vi "to string.vi"(8 "error in":errorcluster, 11 "Instrument configuration":refnum<class "Instrument configuration.lvclass">) -> (0 "error out":errorcluster, 1 "data":string, 2 "version":string, 3 "Instrument configuration out":refnum<class "Instrument configuration.lvclass">)   [LabVIEW 2025, in "Abstract Engine.lvlib" / "Instrument configuration.lvclass"]
doc: "Provides an interface for saving a module configuration to a file or other serialized data source. It is recommended that all children of this class store data in two sets--data required for its own initialization, and any data required for parent initialization--and that each implementation uses the <b>Call Parent Method</b> primitive to serialize parent information.Copyright 2017 National Instruments Corporation\n\nLicensed under the Apache License, Version 2.0 (the \"License\"); you may not use this file except in compliance with the License. You may obtain a copy of the License at http://www.apache.org/licenses/LICENSE-2.0\nUnless required by applicable law or agreed to in writing, software distributed under the License is distributed on an \"AS IS\" BASIS, WITHOUT WARRANTIES OR CONDITIONS OF ANY KIND, either express or implied. See the License for the specific language governing permissions and limitations under the License."
uses:
  Instrument configuration.lvclass
  Instrument configuration.lvclass/Instrument configuration.ctl
  Users/Public/Documents/Sandia National Labs/TSS Plugin/CEF.lvlibp/serializable configuration/CEF_serializable configuration.lvclass
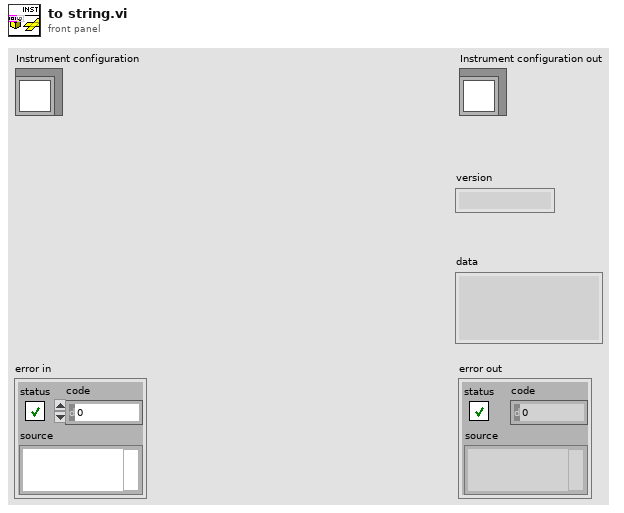
[diagram p1: front panel]
types:
  T1 = typedef "Abstract Engine.lvlib/Instrument configuration.lvclass/Default Instrument.ctl" = cluster{"Type":string, "Engine IP Address":string, "Engine Port":u32, "Address":string, "SW Alias":string, "Description":string, "Enabled":bool, "Model":string, "Serial Number":string, "Asset Number":string, "Calibration Date":string}
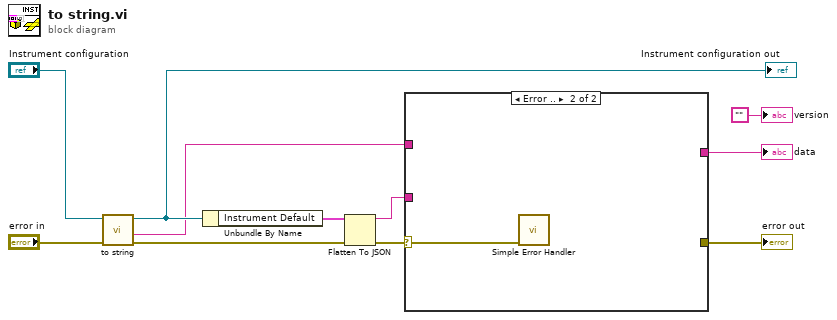
[diagram p0: block diagram]
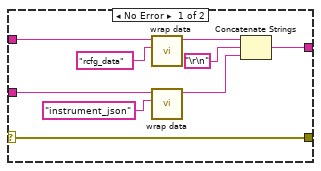
[diagram p2: hidden frame]
diagram:
  n1 = call-parent "to string.vi"("error in"="error in", "CEF_Configuration in"="Instrument configuration") -> ("error out"=w8:errorcluster, "data"=w2:string, "CEF_Configuration out"=w9:refnum<class "Instrument configuration.lvclass">)  [unwired: 6 in, 1 out]
  "Instrument configuration out" <- w9
  n2 = Unbundle By Name(w9) -> ("Instrument Default"=w5:T1)
  n3 = Flatten To JSON(anything=w5, error in (no error)=w8) -> (JSON string=w3:string, 11:w6:errorcluster)  [unwired: 1 in]
  n4 = case shown="Error .." w6 {
    selector: w6 -> [w20 w21]
    tunnel: [w20 _] -> w4
    tunnel: w3 -> [w16 _]
    tunnel: w2 -> [w14 _]
    tunnel: [w12 _] -> w1
    frame No Error {
      n5 = call "wrap data.vi"("identifier"="rcfg_data" ("additional identifier"), "data to wrap"=w14) -> ("wrapped data"=w19:string)  [unwired: 9 in]
      n6 = call "wrap data.vi"("identifier"="instrument_json" ("additional identifier"), "data to wrap"=w16) -> ("wrapped data"=w18:string)  [unwired: 9 in]
      n7 = Concatenate Strings(w19, "\r\n", w18) -> (w12:string)
    }
    frame Error {
      n8 = call <vilib>:"Simple Error Handler.vi"("error in (no error)"=w21) -> ()  [unwired: 4 in, 5 out]
    }
  }
  "error out" <- w4
  "data" <- w1
  "version" <- ""
